vi "testParseStateQueueWhitespaceTest1.vi"(8 "error in (no error)":errorcluster, 11 "testStateMachineUtilities in":refnum<class "testStateMachineUtilities.lvclass">) -> (0 "error out":errorcluster, 3 "testStateMachineUtilities out":refnum<class "testStateMachineUtilities.lvclass">)   [LabVIEW 2013, in "testStateMachineUtilities.lvclass"]
uses:
  testStateMachineUtilities.lvclass
  source/State Machine Support API/Build State String with Arguments.vi
panel:
  out "Array":string[](array[string])
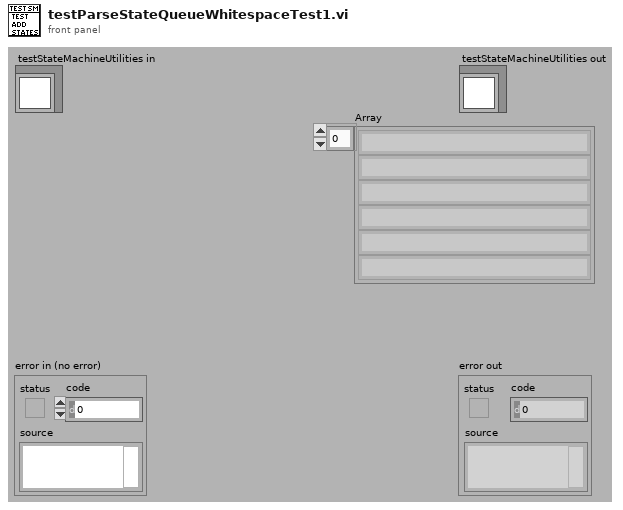
[diagram p1: front panel]
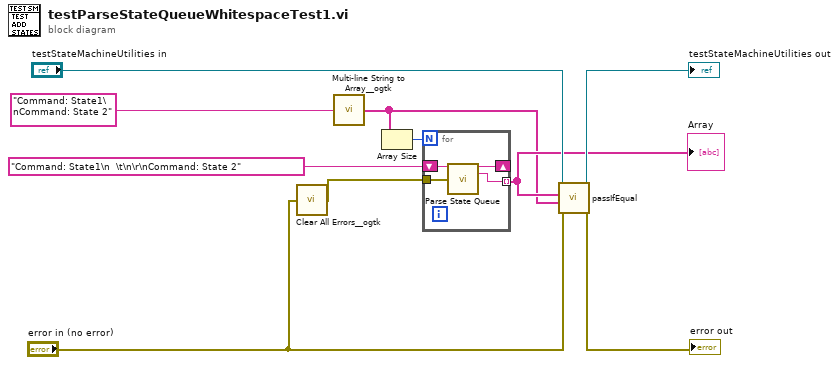
[diagram p0: block diagram]
diagram:
  n1 = call <userlib>:"Clear All Errors__ogtk.vi"("Error In"="error in (no error)") -> ("Error Out"=w6:errorcluster)  [unwired: 3 in]
  n2 = call <userlib>:"Multi-line String to Array__ogtk.vi"("string"="Command: State1\nCommand: State 2" ("State Queue")) -> ("lines"=w3:string[])
  n3 = Array Size(array=w3) -> (size(s)=w4:i32)
  n4 = for {
    N: w4 -> [_]
    tunnel: w6 -> [w13]
    tunnel: [w12] -> w5 mode=indexing
    shift-right: [w11] -> _
    shift-left: "Command: State1\n  \t\n\r\nCommand: State 2" ("State Queue") -> [w14]
    n5 = call "Parse State Queue.vi"("State Queue"=w14, "Error In (no error)"=w13) -> ("Remaining States"=w11:string, "Current State"=w12:string)  [unwired: 11 in, 1 out]
  }
  "Array" <- w5
  n6 = call-dynamic "passIfEqual.vi"("error in (no error)"="error in (no error)", "y"=w3, "x"=w5, "TestCase in"="testStateMachineUtilities in") -> ("error out"=→"error out":errorcluster, "TestCase out"=→"testStateMachineUtilities out":refnum<class "testStateMachineUtilities.lvclass">)  [unwired: 6 in]
